vi "Check For Latched Booleans.vi"(8 "error in":errorcluster, 11 "path of type":path) -> (0 "error out":errorcluster, 3 "path of type out":path)   [LabVIEW 2020, in "Plug-In SDK Measurement.lvlib"]
uses:
  Plug-In SDK Measurement.lvlib
  Error Strings Global Internal.vi
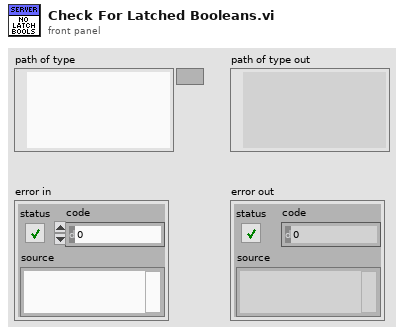
[diagram p1: front panel]
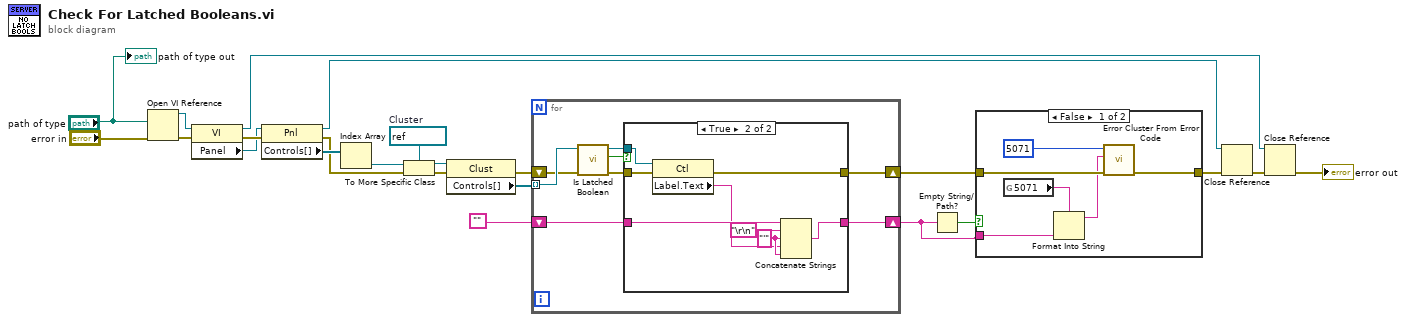
[diagram p0: block diagram]
diagram:
  w23 = refnum<vi> refnum  # Cluster
  n1 = Open VI Reference(vi path="path of type", error in (no error)="error in") -> (vi reference=w11:refnum<vi>, error out=w18:errorcluster)  [unwired: 4 in]
  n2 = property class="VI"(reference=w11, error in=w18) -> (reference out=w15:refnum<vi>, error out=w17:errorcluster, "Panel"=w12:refnum<vi>)
  n3 = property class="Pnl"(reference=w12, error in=w17) -> (reference out=w14:refnum<vi>, error out=w8:errorcluster, "Controls[]"=w13:refnum<vi>[])
  n4 = Index Array(array=w13) -> (element=w10:refnum<vi>)  [unwired: 1 in]
  n5 = To More Specific Class(target class=w23, reference=w10, error in=w8) -> (specific class reference=w22:refnum<vi>, error out=w20:errorcluster)
  n6 = property class="Clust"(reference=w22, error in=w20) -> (error out=w19:errorcluster, "Controls[]"=w21:refnum<vi>[])  [unwired: 1 out]
  n7 = for {
    tunnel: w21 -> [w28] mode=indexing
    shift-right: [w31] -> w5
    shift-left: w19 -> [w27]
    shift-right: [w29] -> w1
    shift-left: "" -> [w30]
    n8 = call "Is Latched Boolean.vi"("error in"=w27, "control in"=w28) -> ("error out"=w24:errorcluster, "is latched boolean"=w25:bool, "control out"=w26:refnum<vi>)  [unwired: 7 in]
    n9 = case shown="True" w25 {
      tunnel: [w32 w36] -> w31
      tunnel: w30 -> [w33 w40]
      tunnel: [w33 w41] -> w29
      tunnel: w26 -> [_ w37]
      tunnel: w24 -> [w32 w34]
      frame False {
      }
      frame True {
        w38 = "'" ("string")
        n10 = property class="Ctl"(reference=w37, error in=w34) -> (error out=w36:errorcluster, "Label.Text"=w35:string)  [unwired: 1 out]
        n11 = Concatenate Strings(w40, "\r\n", w38, w35, w38) -> (w41:string)
      }
    }
  }
  n12 = Empty String/Path?(string/path=w1) -> (empty?=w2:bool)
  n13 = case shown="False" w2 {
    tunnel: w5 -> [w46 w48]
    tunnel: [w45 w48] -> w4
    tunnel: w1 -> [w43 _]
    frame False {
      n14 = global read "Error Strings Global Internal.vi" "5071"() -> (w44:string)
      n15 = Format Into String(format string=w44, w43) -> (resulting string=w42:string)  [unwired: 2 in, 1 out]
      n16 = call <vilib>:"Error Cluster From Error Code.vi"("error in (no error)"=w46, "error message (\"\")"=w42, "error code (0)"=5071) -> ("error out"=w45:errorcluster)  [unwired: 6 in]
    }
    frame True {
    }
  }
  n17 = Close Reference(reference=w14, error in (no error)=w4) -> (error out=w16:errorcluster)
  n18 = Close Reference(reference=w15, error in (no error)=w16) -> (error out=→"error out":errorcluster)
  "path of type out" <- "path of type"
